vi "GetControlValues.vi"(5 "As List":bool, 7 "UseEnum (true)":bool=TRUE, 8 "error in":errorcluster, 11 "ControlList":string) -> (0 "error out":errorcluster, 3 "Control Values":string)   [LabVIEW 2019]
panel:
  # "先頭行がvi名\n次行からがctrl名\n空行を挟んで次のvi名\nvi名やctrl名は | で区切って後ろに表示名を指定可能\nJSON中には表示名が現れる\n// から始まる行はコメントとして無視される"
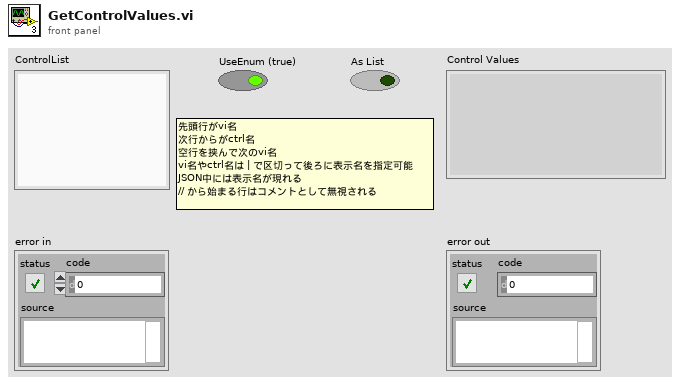
[diagram p1: front panel]
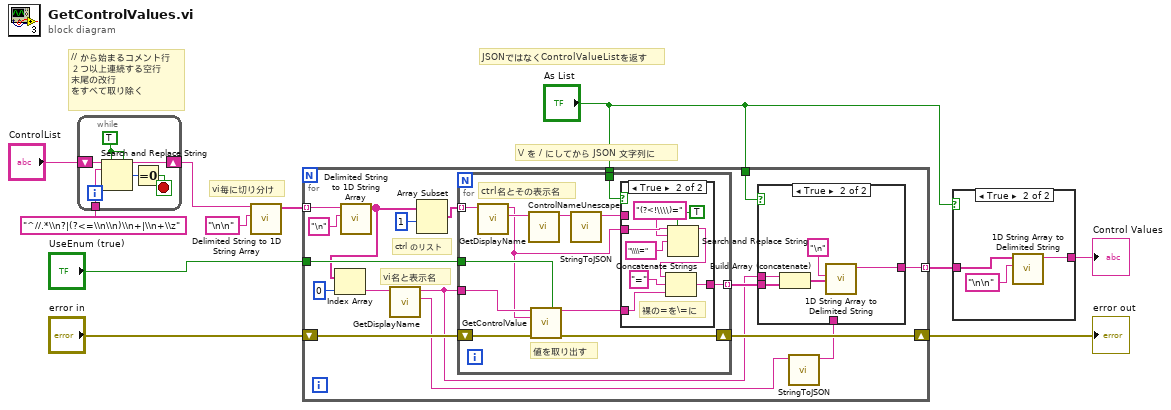
[diagram p0: block diagram]
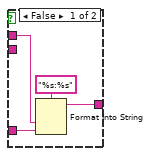
[diagram p2: hidden frame]
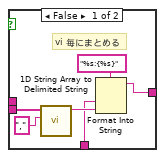
[diagram p3: hidden frame]
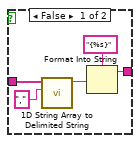
[diagram p4: hidden frame]
diagram:
  # "JSONではなくControlValueListを返す"
  # "// から始まるコメント行\n２つ以上連続する空行\n末尾の改行\nをすべて取り除く"
  # "\\/ を / にしてから JSON 文字列に"
  # "vi毎に切り分け"
  n1 = while {
    shift-right: [w17] -> w2
    shift-left: "ControlList" -> [w15]
    tunnel: "^//.*\\n?|(?<=\\n\\n)\\n+|\\n+\\z" ("search string") -> [w12]
    stop <- w13 stop-if-true
    w16 = TRUE ("multiline? (F)")
    n2 = Search and Replace String(replace all?=w16, multiline?=w16, input string=w15, search string=w12) -> (result string=w17:string, number of replacements=w14:i32)  [unwired: 4 in, 2 out]
    n3 = Equal To 0?(x=w14) -> (x = 0?=w13:bool)
  }
  n4 = call <vilib>:"Delimited String to 1D String Array.vi"("delimiter"="\n\n", "delimited string"=w2) -> ("string array"=w5:string[])  [unwired: 9 in]
  n5 = for {
    tunnel: w5 -> [w22] mode=indexing
    tunnel: [w28] -> w10 mode=indexing
    tunnel: "UseEnum (true)" -> [w31]
    shift-right: [w26] -> w6
    shift-left: "error in" -> [w27]
    tunnel: "As List" -> [w20]
    tunnel: "As List" -> [w19]
    # "vi名と表示名"
    # "ctrl のリスト"
    n6 = call <vilib>:"Delimited String to 1D String Array.vi"("delimiter"="\n", "delimited string"=w22) -> ("string array"=w21:string[])  [unwired: 9 in]
    n7 = Index Array(array=w21, index=0) -> (element=w29:string)
    n8 = call "GetDisplayName.vi"("Name in"=w29) -> ("Display Name"=w25:string, "Name"=w18:string)  [unwired: 9 in]
    n9 = Array Subset(array=w21, index=1) -> (w32:string[])  [unwired: 1 in]
    n10 = for {
      tunnel: w32 -> [w46] mode=indexing
      tunnel: w18 -> [w43]
      tunnel: w31 -> [w42]
      shift-right: [w40] -> w26
      shift-left: w27 -> [w44]
      tunnel: [w45] -> w30 mode=indexing
      tunnel: w20 -> [w36]
      # "値を取り出す"
      # "ctrl名とその表示名"
      n11 = call "GetDisplayName.vi"("Name in"=w46) -> ("Display Name"=w38:string, "Name"=w35:string)  [unwired: 9 in]
      n12 = call "ControlNameUnescape.vi"("escaped string"=w38) -> ("label"=w37:string)  [unwired: 10 in]
      n13 = call "GetControlValue.vi"("vi"=w43, "UseEnum (true)"=w42, "ctrl"=w35, "error in (no error)"=w44) -> ("String out"=w41:string, "error out"=w40:errorcluster)  [unwired: 9 in, 1 out]
      n14 = call "StringToJSON.vi"("input text"=w37) -> ("JSON string"=w39:string)  [unwired: 10 in]
      n15 = case shown="True" w36 {
        tunnel: [w49 w58] -> w45
        tunnel: w41 -> [w48 w56]
        tunnel: w39 -> [w47 _]
        tunnel: w35 -> [_ w55]
        frame False {
          n16 = Format Into String(format string="%s:%s", w47, w48) -> (resulting string=w49:string)  [unwired: 2 in, 1 out]
        }
        frame True {
          # "裸の=を\\=に"
          n17 = Search and Replace String(replace all?=TRUE ("replace all? (F)"), input string=w55, search string="(?<!\\\\)=" ("substring (\"\")"), replace string="\\\\=" ("replace string (\"\")")) -> (result string=w52:string)  [unwired: 4 in, 3 out]
          n18 = Concatenate Strings(w52, "=" ("string"), w56) -> (w58:string)
        }
      }
    }
    n19 = call "StringToJSON.vi"("input text"=w25) -> ("JSON string"=w24:string)  [unwired: 10 in]
    n20 = case shown="True" w19 {
      tunnel: w30 -> [w62 w69]
      tunnel: [w60 w66] -> w28
      tunnel: w24 -> [w59 _]
      tunnel: w18 -> [_ w65]
      frame False {
        # "vi 毎にまとめる"
        n21 = call <vilib>:"1D String Array to Delimited String.vi"("delimiter"=",", "string array"=w62) -> ("delimited string"=w61:string)  [unwired: 9 in]
        n22 = Format Into String(format string="%s:{%s}", w59, w61) -> (resulting string=w60:string)  [unwired: 2 in, 1 out]
      }
      frame True {
        n23 = Build Array (concatenate)(w65, w69) -> (w67:string[])
        n24 = call <vilib>:"1D String Array to Delimited String.vi"("delimiter"="\n" ("string"), "string array"=w67) -> ("delimited string"=w66:string)  [unwired: 9 in]
      }
    }
  }
  "error out" <- w6
  n25 = case shown="True" "As List" {
    tunnel: w10 -> [w74 w77]
    tunnel: [w70 w75] -> w8
    frame False {
      n26 = call <vilib>:"1D String Array to Delimited String.vi"("delimiter"=",", "string array"=w74) -> ("delimited string"=w72:string)  [unwired: 9 in]
      n27 = Format Into String(format string="{%s}", w72) -> (resulting string=w70:string)  [unwired: 2 in, 1 out]
    }
    frame True {
      n28 = call <vilib>:"1D String Array to Delimited String.vi"("delimiter"="\n\n" ("string"), "string array"=w77) -> ("delimited string"=w75:string)  [unwired: 9 in]
    }
  }
  "Control Values" <- w8
